vi "Processing.Stop.vi"(8 "error in (no error)":errorcluster) -> (0 "error out":errorcluster)   [LabVIEW 2019, in "Tools.lvlib"]
uses:
  Tools.lvlib
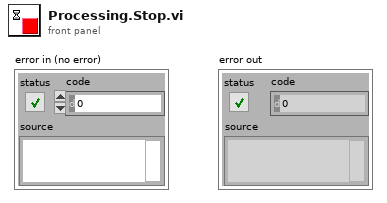
[diagram p1: front panel]
types:
  T1 = enum32{"Bad", "Idle", "Run top level", "Running"}
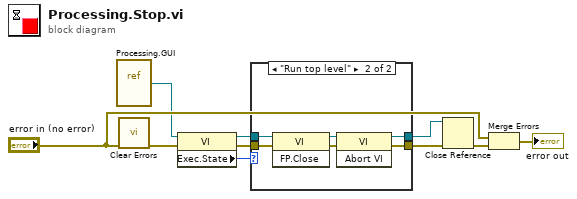
[diagram p0: block diagram]
diagram:
  n1 = vi-ref "Processing.GUI.vi"() -> (w3:refnum<vi>)
  n2 = call <vilib>:"Clear Errors.vi"("error in (no error)"="error in (no error)") -> ("error out"=w7:errorcluster)  [unwired: 5 in, 1 out]
  n3 = property class="VI"(reference=w3, error in=w7) -> (reference out=w2:refnum<vi>, error out=w4:errorcluster, "Exec.State"=w1:T1)
  n4 = case shown="\"Run top level\"" w1 {
    tunnel: [w11 w16] -> w10
    tunnel: [w12 w15] -> w9
    tunnel: w4 -> [w11 w14]
    tunnel: w2 -> [w12 w13]
    frame Default {
    }
    frame "Run top level" {
      n5 = invoke class="VI" method="FP.Close"(reference=w13, error in=w14) -> (reference out=w18:refnum<vi>, error out=w17:errorcluster)  [unwired: 1 in, 1 out]
      n6 = invoke class="VI" method="Abort VI"(reference=w18, error in=w17) -> (reference out=w15:refnum<vi>, error out=w16:errorcluster)  [unwired: 1 in, 1 out]
    }
  }
  n7 = Close Reference(reference=w9, error in (no error)=w10) -> (error out=w8:errorcluster)
  n8 = Merge Errors("error in (no error)", w8) -> (→"error out":errorcluster)
